vi "create.vi"(8 "error in (no error)":errorcluster) -> (0 "error out":errorcluster, 3 "Banking Transactions out":refnum<class "BankingTransactionList.lvclass">)   [LabVIEW 2018, in "BankingTransactionList.lvclass"]
uses:
  BankingTransactionList.lvclass
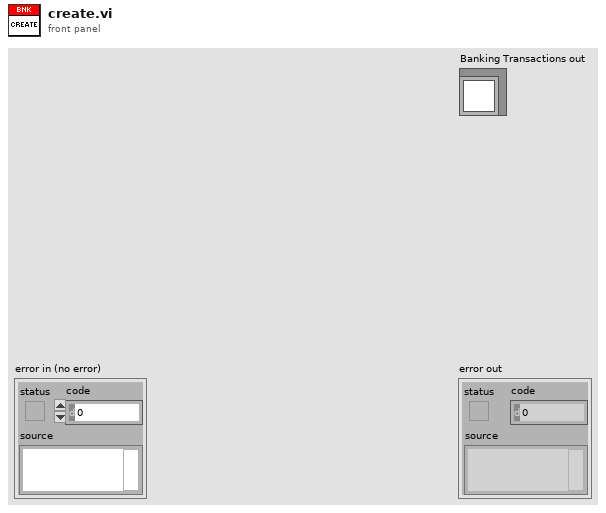
[diagram p1: front panel]
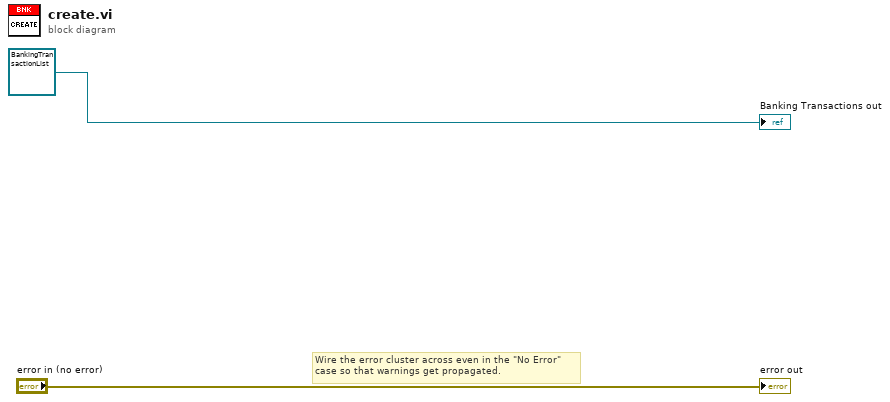
[diagram p0: block diagram]
diagram:
  # "Wire the error cluster across even in the \"No Error\"\ncase so that warnings get propagated."
  "error out" <- "error in (no error)"
  "Banking Transactions out" <- refnum<class "BankingTransactionList.lvclass"> refnum ("Banking Transactions in")
